vi "CThread Send Terminate Signal.vi"(0 "Terminate":bool=TRUE caption="Terminate? (T)") -> ()   [LabVIEW 2012, in "CThread.lvlib"]
uses:
  CThread.lvlib
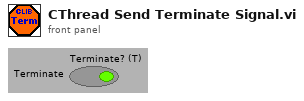
[diagram p1: front panel]
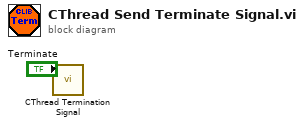
[diagram p0: block diagram]
diagram:
  n1 = call "CThread Termination Signal.vi"("Send Term Signal?"="Terminate") -> ()  [unwired: 4 in, 1 out]
